vi "Open TCP Connection.vi"(2 "TCP Port":u16=12344, 3 "timeout ms (60000)":i32=60000, 4 "Name of RT target":string) -> (0 "error out":errorcluster, 1 "connection ID":refnum<k5>)   [LabVIEW 2013]
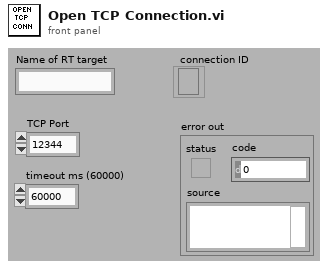
[diagram p1: front panel]
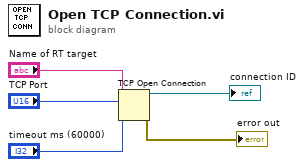
[diagram p0: block diagram]
diagram:
  n1 = TCP Open Connection(address="Name of RT target", remote port or service name="TCP Port", timeout ms (60000)="timeout ms (60000)") -> (connection ID=→"connection ID":refnum<k5>, error out=→"error out":errorcluster)  [unwired: 1 in, 1 out]
